vi "gen_time_array.vi"(11 "Acquisition Settings":T1) -> (3 "Time Out":dbl[](array[numeric]))   [LabVIEW 2016]
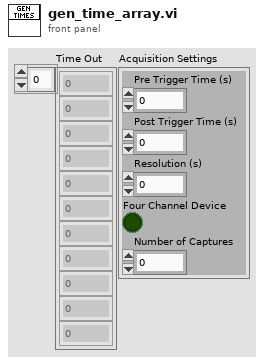
[diagram p1: front panel]
types:
  T1 = cluster{"Pre Trigger Time (s)":dbl, "Post Trigger Time (s)":dbl, "Resolution (s)":dbl, "Four Channel Device":bool, "Number of Captures":dbl}
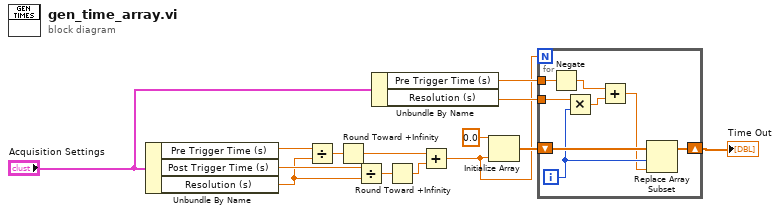
[diagram p0: block diagram]
diagram:
  n1 = Unbundle By Name("Acquisition Settings") -> ("Pre Trigger Time (s)"=w13:dbl, "Post Trigger Time (s)"=w14:dbl, "Resolution (s)"=w12:dbl)
  n2 = Divide(x=w13, y=w12) -> (x/y=w11:dbl)
  n3 = Round Toward +Infinity(x=w11) -> (ceil(x): smallest int >= x=w8:dbl)
  n4 = Divide(x=w14, y=w12) -> (x/y=w10:dbl)
  n5 = Unbundle By Name("Acquisition Settings") -> ("Pre Trigger Time (s)"=w5:dbl, "Resolution (s)"=w4:dbl)
  n6 = Round Toward +Infinity(x=w10) -> (ceil(x): smallest int >= x=w9:dbl)
  n7 = Add(x=w8, y=w9) -> (x+y=w2:dbl)
  n8 = Initialize Array(0.0 ("element"), w2) -> (w6:dbl[])
  n9 = for {
    N: w2 -> [_]
    shift-right: [w21] -> w3
    shift-left: w6 -> [w22]
    tunnel: w5 -> [w20]
    tunnel: w4 -> [w16]
    i -> [w18]
    n10 = Negate(x=w20) -> (-x=w19:dbl)
    n11 = Multiply(x=w16, y=w18) -> (x*y=w17:dbl)
    n12 = Add(x=w19, y=w17) -> (x+y=w15:dbl)
    n13 = Replace Array Subset(array=w22, new element=w15, index=w18) -> (w21:dbl[])
  }
  "Time Out" <- w3
